vi "RSB.vi"(2 "R":bool[](array[boolean]), 3 "S":bool[](array[boolean])) -> (0 "~Q":bool[](array[boolean]), 1 "Q":bool[](array[boolean]))   [LabVIEW 2019, in "Triggers.lvlib"]
uses:
  Triggers.lvlib
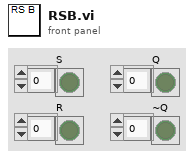
[diagram p1: front panel]
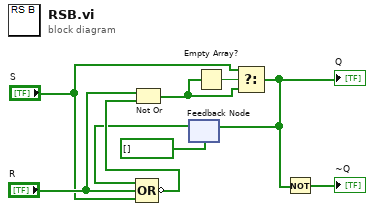
[diagram p0: block diagram]
diagram:
  n1 = feedback #1(bool[] [] ("S")) -> (w7:bool[])
  n2 = Compound Arithmetic op=OR(w7, "R", "S") -> (invert w8:bool[])
  n3 = Not Or(1:w8, 2:"R") -> (0:w4:bool[])
  n4 = Empty Array?(array=w4) -> (empty?=w5:bool)
  n5 = Select(t="S", s=w5, f=w4) -> (s? t:f=w3:bool[])
  "Q" <- w3
  n6 = feedback-in #1(w3) -> ()
  n7 = Not(x=w3) -> (.not. x?=→"~Q":bool[])
